vi "TalonFXSSetter.vi"   [LabVIEW 2023]
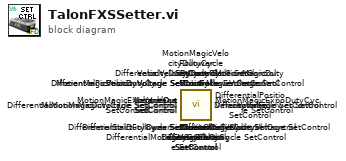
[diagram p0: block diagram]
diagram:
  n1 = call <vilib>:"DynamicMotionMagicVoltage SetControl.vi"() -> ()  [unwired: 26 in, 2 out]
  n2 = call <vilib>:"DynamicMotionMagicDutyCycle SetControl.vi"() -> ()  [unwired: 26 in, 2 out]
  n3 = call <vilib>:"MotionMagicExpoVoltage SetControl.vi"() -> ()  [unwired: 26 in, 2 out]
  n4 = call <vilib>:"MotionMagicExpoDutyCycle SetControl.vi"() -> ()  [unwired: 26 in, 2 out]
  n5 = call <vilib>:"MotionMagicVelocityVoltage SetControl.vi"() -> ()  [unwired: 26 in, 2 out]
  n6 = call <vilib>:"MotionMagicVelocityDutyCycle SetControl.vi"() -> ()  [unwired: 26 in, 2 out]
  n7 = call <vilib>:"StaticBrake SetControl.vi"() -> ()  [unwired: 26 in, 2 out]
  n8 = call <vilib>:"CoastOut SetControl.vi"() -> ()  [unwired: 26 in, 2 out]
  n9 = call <vilib>:"NeutralOut SetControl.vi"() -> ()  [unwired: 26 in, 2 out]
  n10 = call <vilib>:"DifferentialStrictFollower SetControl.vi"() -> ()  [unwired: 26 in, 2 out]
  n11 = call <vilib>:"DifferentialFollower SetControl.vi"() -> ()  [unwired: 26 in, 2 out]
  n12 = call <vilib>:"StrictFollower SetControl.vi"() -> ()  [unwired: 26 in, 2 out]
  n13 = call <vilib>:"Follower SetControl.vi"() -> ()  [unwired: 26 in, 2 out]
  n14 = call <vilib>:"DifferentialMotionMagicVoltage SetControl.vi"() -> ()  [unwired: 26 in, 2 out]
  n15 = call <vilib>:"DifferentialMotionMagicDutyCycle SetControl.vi"() -> ()  [unwired: 26 in, 2 out]
  n16 = call <vilib>:"DifferentialVelocityVoltage SetControl.vi"() -> ()  [unwired: 26 in, 2 out]
  n17 = call <vilib>:"DifferentialVelocityDutyCycle SetControl.vi"() -> ()  [unwired: 26 in, 2 out]
  n18 = call <vilib>:"DifferentialPositionVoltage SetControl.vi"() -> ()  [unwired: 26 in, 2 out]
  n19 = call <vilib>:"DifferentialPositionDutyCycle SetControl.vi"() -> ()  [unwired: 26 in, 2 out]
  n20 = call <vilib>:"DifferentialVoltage SetControl.vi"() -> ()  [unwired: 26 in, 2 out]
  n21 = call <vilib>:"DifferentialDutyCycle SetControl.vi"() -> ()  [unwired: 26 in, 2 out]
  n22 = call <vilib>:"MotionMagicVoltage SetControl.vi"() -> ()  [unwired: 26 in, 2 out]
  n23 = call <vilib>:"MotionMagicDutyCycle SetControl.vi"() -> ()  [unwired: 26 in, 2 out]
  n24 = call <vilib>:"VelocityVoltage SetControl.vi"() -> ()  [unwired: 26 in, 2 out]
  n25 = call <vilib>:"VelocityDutyCycle SetControl.vi"() -> ()  [unwired: 26 in, 2 out]
  n26 = call <vilib>:"PositionVoltage SetControl.vi"() -> ()  [unwired: 26 in, 2 out]
  n27 = call <vilib>:"PositionDutyCycle SetControl.vi"() -> ()  [unwired: 26 in, 2 out]
  n28 = call <vilib>:"VoltageOut SetControl.vi"() -> ()  [unwired: 26 in, 2 out]
  n29 = call <vilib>:"DutyCycleOut SetControl.vi"() -> ()  [unwired: 26 in, 2 out]
